vi "read text file advanced.vi"() -> ()   [LabVIEW 2016]
panel:
  out "File Contents":string
  out "File Size (in bytes)":i64
  in  "Path":path
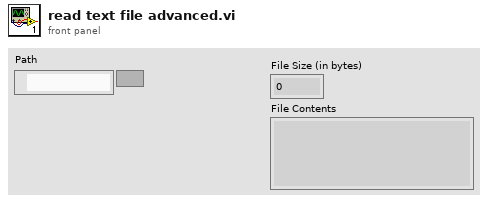
[diagram p1: front panel]
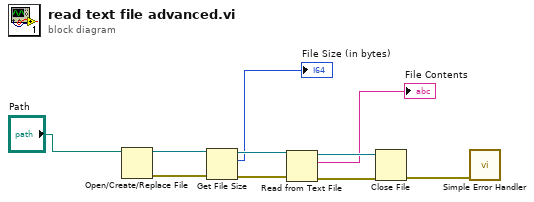
[diagram p0: block diagram]
diagram:
  n1 = Open/Create/Replace File(file path (use dialog)="Path") -> (refnum out=w9:refnum<file>, error out=w6:errorcluster)  [unwired: 5 in, 1 out]
  n2 = Get File Size(file=w9, error in=w6) -> (refnum out=w8:refnum<file>, size (in bytes)=→"File Size (in bytes)":i64, 0:w5:errorcluster)
  n3 = Read from Text File(file (use dialog)=w8, error in=w5) -> (refnum out=w7:refnum<file>, text=→"File Contents":string, error out=w4:errorcluster)  [unwired: 2 in, 1 out]
  n4 = Close File(refnum=w7, error in=w4) -> (error out=w3:errorcluster)  [unwired: 1 out]
  n5 = call <vilib>:"Simple Error Handler.vi"("error in (no error)"=w3) -> ()  [unwired: 4 in, 5 out]
